vi "UWB Serial Write.vi"(6 "String":string="*IDN?\n", 8 "error in (no error)":errorcluster, 9 "FPGA Interface":refnum<k20>) -> (2 "error out":errorcluster, 3 "FPGA Interface Out":refnum<k20>)   [LabVIEW 2016]
uses:
  <vilib>/Utility/error.llb/Error Cluster From Error Code.vi
  <vilib>/rvi/errors/niLvFpgaAdjustHostInterfaceError.vi
  <vilib>/rvi/interface/nirviReadWriteControl/nirviReadWriteControl.xnode
  NiFpgaLv.dll
  <vilib>/rvi/interface/Simulation/niFpgaSimulationCallBeginRW.vi
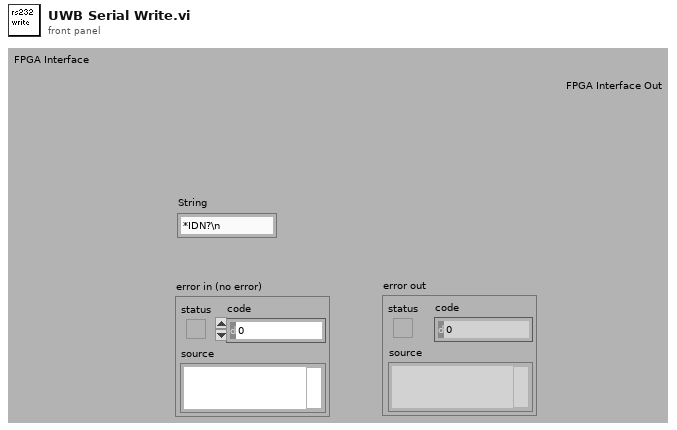
[diagram p1: front panel]
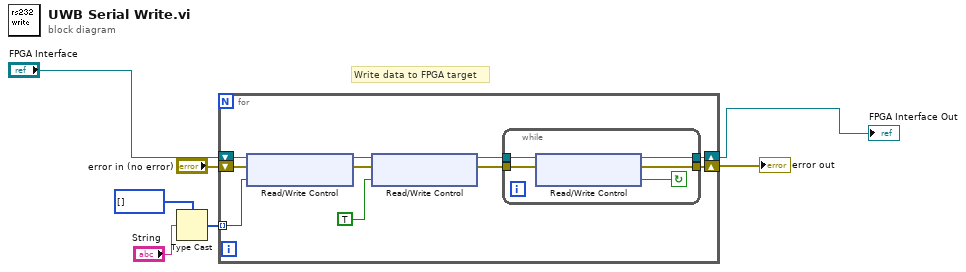
[diagram p0: block diagram]
diagram:
  # "Write data to FPGA target"
  n1 = Type Cast(type=u8[] [], x="String") -> (*(type *) &x=w4:u8[])
  n2 = for {
    tunnel: w4 -> [w15] mode=indexing
    shift-right: [w9] -> w2
    shift-left: "FPGA Interface" -> [w14]
    shift-right: [w8] -> w3
    shift-left: "error in (no error)" -> [w13]
    n3 = xnode "Read/Write Control"("FPGA VI Reference In"=w14, "error in"=w13, "Write: UWB Char"=w15) -> ("FPGA VI Reference Out"=w17:refnum<k20>, "error out"=w16:errorcluster)
    n4 = xnode "Read/Write Control"("FPGA VI Reference In"=w17, "error in"=w16, "Write: UWB Data"=TRUE ("Data Read")) -> ("FPGA VI Reference Out"=w11:refnum<k20>, "error out"=w10:errorcluster)
    n5 = while {
      tunnel: w11 -> [w22]
      tunnel: w10 -> [w21]
      tunnel: [w20] -> w9
      tunnel: [w19] -> w8
      stop <- w18 continue-if-true
      n6 = xnode "Read/Write Control"("FPGA VI Reference In"=w22, "error in"=w21) -> ("FPGA VI Reference Out"=w20:refnum<k20>, "error out"=w19:errorcluster, "Write: UWB Data"=w18:bool)
    }
  }
  "error out" <- w3
  "FPGA Interface Out" <- w2
